vi "Button Rising Edge Toggle.vi"(11 "Button":bool) -> (3 "Rising edge?":bool)   [LabVIEW 2019, in "Joysticks.lvlib" / "Joysticks.lvclass"]
doc: "This VI takes a boolean input and returns a TRUE whenever it sees a rising edge (compared to the last value).\nIt filters continous TRUE values coming from the joystick.\nPlease not this is a reentrant VI, so each instance has its separate memory."
uses:
  Joysticks.lvclass
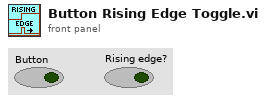
[diagram p1: front panel]
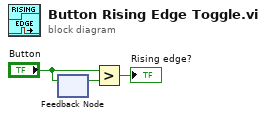
[diagram p0: block diagram]
diagram:
  n1 = feedback #1() -> (w1:bool)  [unwired: 1 in]
  n2 = feedback-in #1("Button") -> ()
  n3 = Greater?(x="Button", y=w1) -> (0:→"Rising edge?":bool)
